vi "DCMotors1.vi"(8 "error in":errorcluster, 9 "Motors Renum":cluster{"Num":i32, "Directly":bool, "KM":dbl}[](array[cluster])=[{"Num"=1, "Directly"=TRUE, "KM"=0.97}, {"Num"=3, "Directly"=FALSE, "KM"=1.0}, {"Num"=0, "Directly"=FALSE, "KM"=0.98}, {"Num"=2, "Directly"=TRUE, "KM"=1.0}], 10 "Input":dbl[](array[slide])=[0.0, 0.0, -0.01, 0.0] step=1.0 scale=-100.0..100.0, 11 "CAN in":refnum<class "CAN.lvclass">) -> (0 "error out":errorcluster, 3 "CAN out":refnum<class "CAN.lvclass">)   [LabVIEW 2020]
uses:
  <vilib>/High Genius/HG_WSI_Tookit/Dependencies/Library/CAN/CAN.lvclass
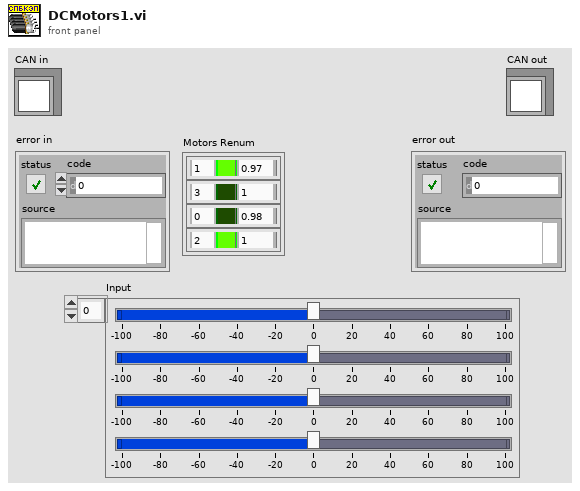
[diagram p1: front panel]
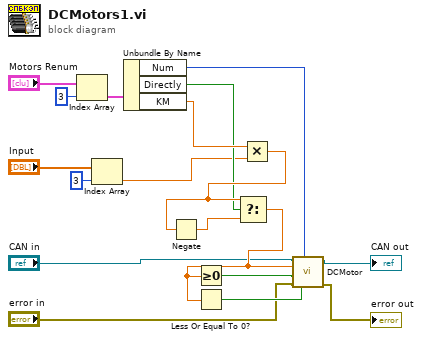
[diagram p0: block diagram]
diagram:
  n1 = Index Array(array="Motors Renum", index=3) -> (element=w7:cluster{"Num":i32, "Directly":bool, "KM":dbl})
  n2 = Index Array(array="Input", index=3) -> (element=w1:dbl)
  n3 = Unbundle By Name(w7) -> ("Num"=w4:i32, "Directly"=w5:bool, "KM"=w6:dbl)
  n4 = Multiply(x=w6, y=w1) -> (x*y=w18:dbl)
  n5 = Negate(x=w18) -> (-x=w14:dbl)
  n6 = Select(t=w18, s=w5, f=w14) -> (s? t:f=w17:dbl)
  n7 = Greater Or Equal To 0?(x=w17) -> (x >= 0?=w15:bool)
  n8 = Less Or Equal To 0?(x=w17) -> (x <= 0?=w16:bool)
  n9 = call "DCMotor.vi"("INB"=w16, "PWM"=w4, "error in (no error)"="error in", "INA"=w15, "Duty Cycle"=w17, "CAN in"="CAN in") -> ("error out"=→"error out":errorcluster, "CAN out"=→"CAN out":refnum<class "CAN.lvclass">)  [unwired: 4 in]
